vi "Get UI Ref.vi"(8 "error in (no error)":errorcluster, 11 "9224 in":refnum<class "9224.lvclass">) -> (0 "error out":errorcluster, 1 "Show SubPanel?":bool, 2 "VI Refnum":refnum<vi>, 3 "9224 out":refnum<class "9224.lvclass">)   [LabVIEW 2017, in "Modules.lvlib" / "9224.lvclass"]
uses:
  9224.lvclass
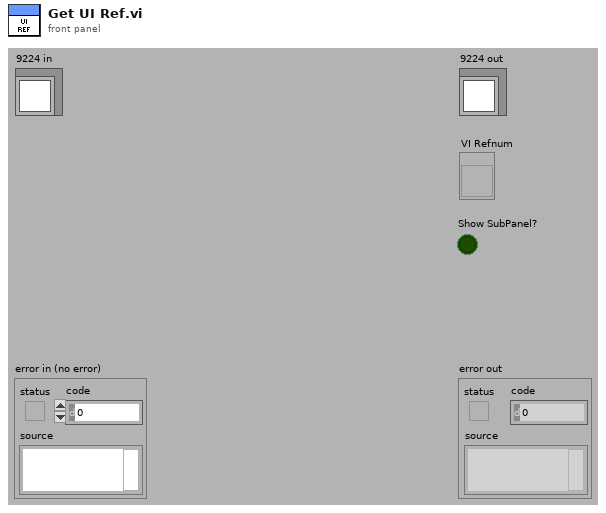
[diagram p1: front panel]
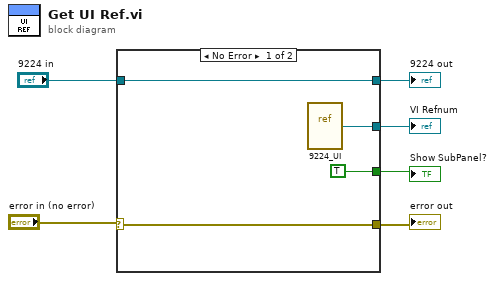
[diagram p0: block diagram]
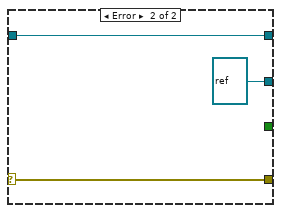
[diagram p2: hidden frame]
diagram:
  n1 = case shown="No Error" "error in (no error)" {
    selector: "error in (no error)" -> [w10 w13]
    tunnel: [w10 w13] -> w5
    tunnel: [w9 refnum<vi> refnum] -> w4
    tunnel: [TRUE _] -> w3
    tunnel: [w7 w11] -> w2
    tunnel: "9224 in" -> [w7 w11]
    frame No Error {
      n2 = vi-ref "9224_UI.vi"() -> (w9:refnum<vi>)
    }
    frame Error {
    }
  }
  "error out" <- w5
  "9224 out" <- w2
  "VI Refnum" <- w4
  "Show SubPanel?" <- w3
